vi "Global Tace.vi"() -> ()   [LabVIEW 2023, in "GUI.lvlib"]
uses:
  GUI.lvlib
panel:
  in  "Trace":string[][](array[string])
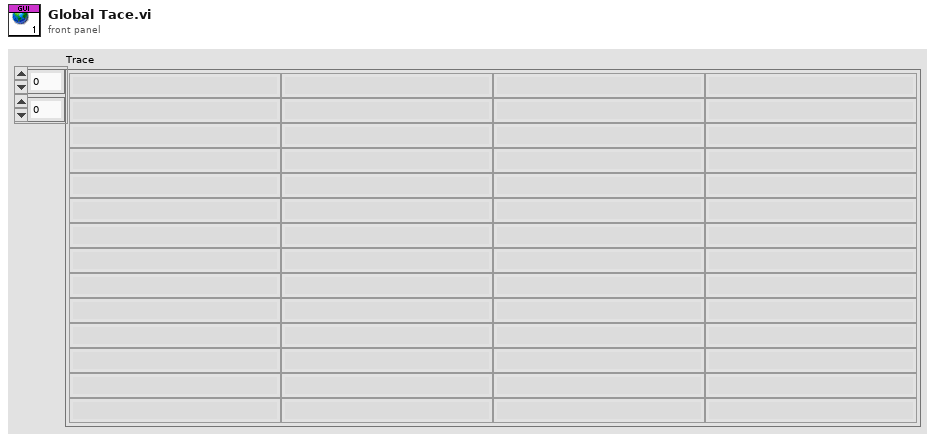
[diagram p1: front panel]
diagram:
